vi "prompt_the_user_but_do_not_linger_v1.0.vi"() -> ()   [LabVIEW 2025]
doc: "Proof of concept/example VI for demonstration.\n\nMichael Panganiban\nSr. Hardware Test Engineer\nFresh Consulting, Inc."
uses:
  controls/home_navigation_btn.ctl
  controls/equipment_navigation_btn.ctl
  controls/settings_navigation_btn.ctl
  controls/test_plan_navigation_btn.ctl
panel:
  in  "test_plan":T1
  in  "settings":T2
  in  "equipment":T3
  in  "home":T4
  in  "Tab":T5(tab)
  out "start_of_test_status":string
  in  "start_test":bool
  # "v1.0.0.1"
  # "HOME"
  # "EQUIPMENT"
  # "SETTINGS"
  # "TEST PLAN CREATION"
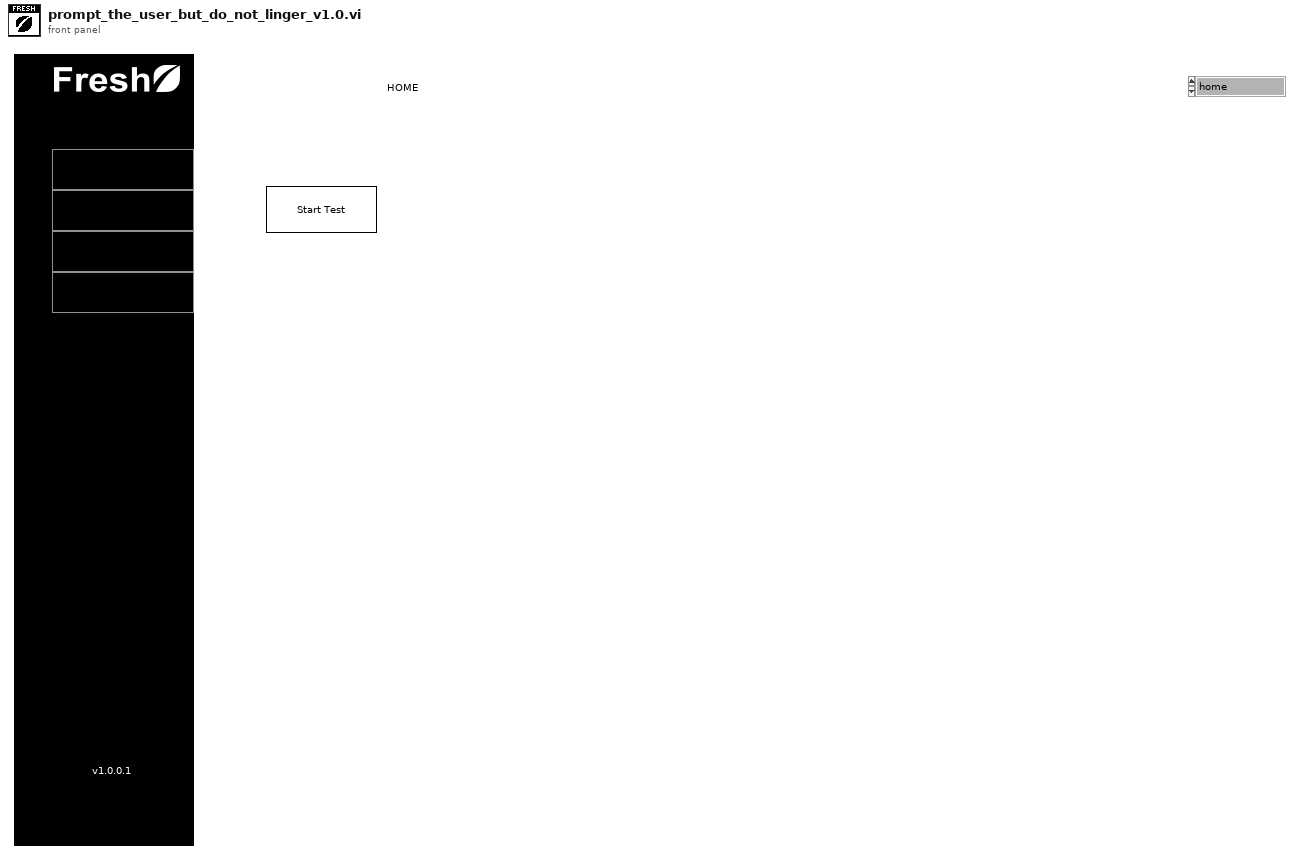
[diagram p1: front panel]
types:
  T1 = typedef "test_plan_navigation_btn.ctl" = bool
  T2 = typedef "settings_navigation_btn.ctl" = bool
  T3 = typedef "equipment_navigation_btn.ctl" = bool
  T4 = typedef "home_navigation_btn.ctl" = bool
  T5 = enum32{"home", "equipment", "settings", "test_plan"}
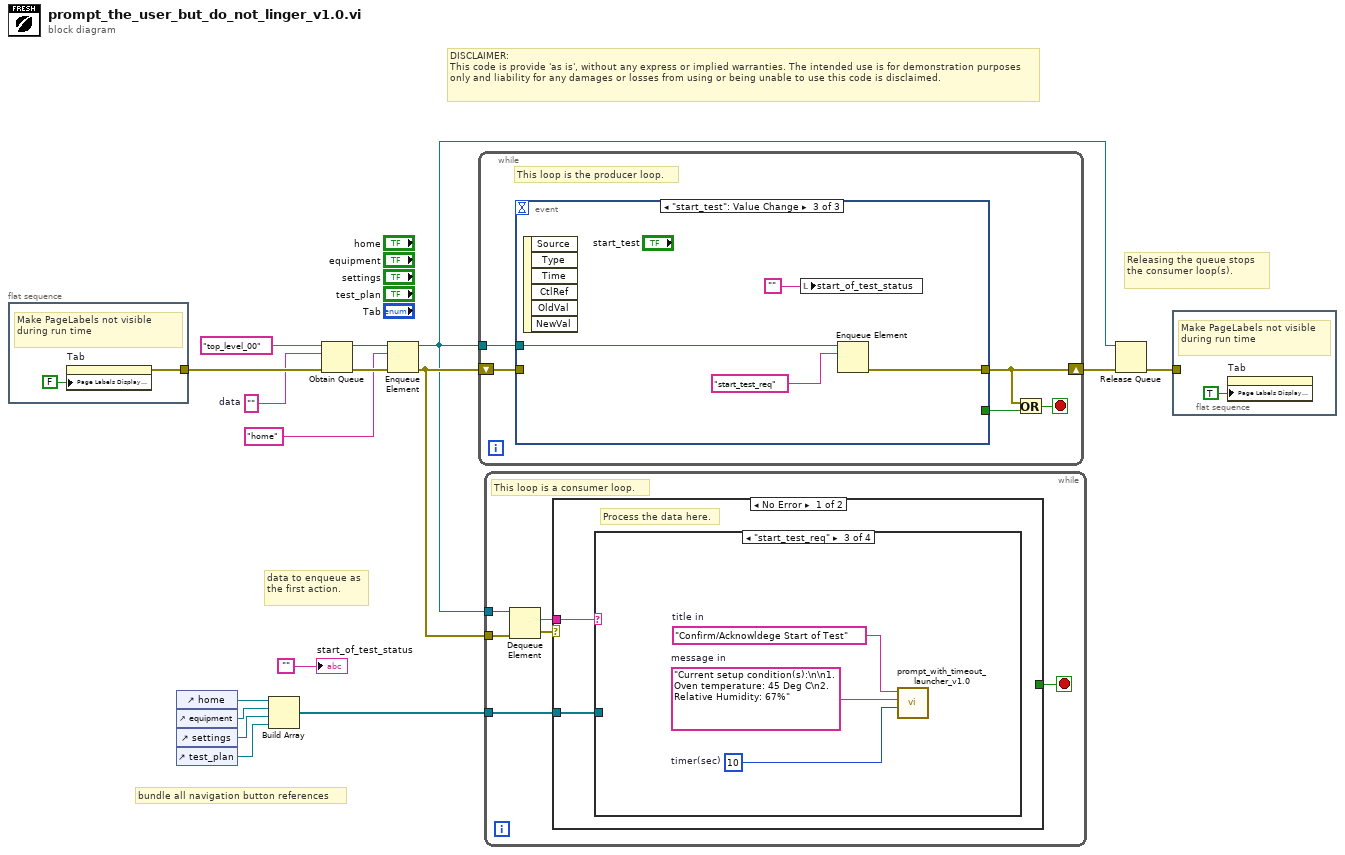
[diagram p0: block diagram]
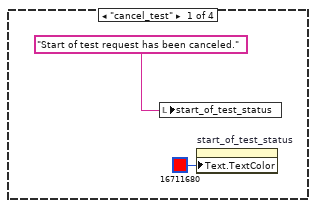
[diagram p2: hidden frame]
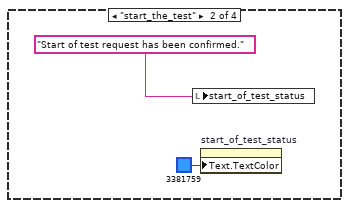
[diagram p3: hidden frame]
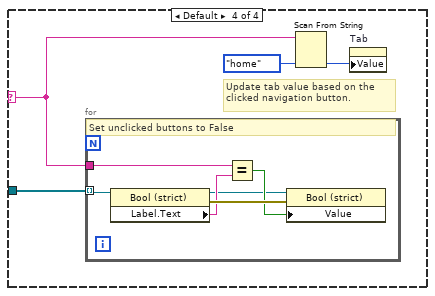
[diagram p4: hidden frame]
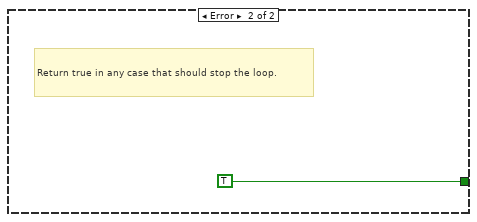
[diagram p5: hidden frame]
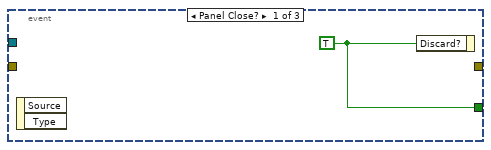
[diagram p6: hidden frame]
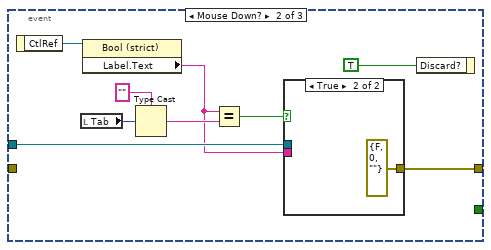
[diagram p7: hidden frame]
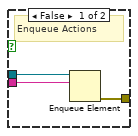
[diagram p8: hidden frame]
diagram:
  w2 = ""  # data
  # "data to enqueue as the first action."
  # "bundle all navigation button references"
  # "DISCLAIMER:\nThis code is provide 'as is', without any express or implied warranties. The intended use is for demonstration purposes only and liability for any damages or losses from using or being unable to use this code is disclaimed."
  # "Releasing the queue stops the consumer loop(s)."
  n1 = flat-sequence {
    tunnel: [w17] -> w15
    frame #0 {
      # "Make PageLabels not visible during run time"
      n2 = property on="Tab" class="TabCtl (strict)"("Page Labels Display Visible?"=FALSE) -> (error out=w17:errorcluster)  [unwired: 2 in, 1 out]
    }
  }
  n3 = control-ref of="home"() -> (w7:refnum<vi>)
  n4 = control-ref of="equipment"() -> (w13:refnum<vi>)
  n5 = control-ref of="settings"() -> (w12:refnum<vi>)
  n6 = control-ref of="test_plan"() -> (w11:refnum<vi>)
  n7 = Build Array(w7, w13, w12, w11) -> (w10:refnum<vi>[])
  n8 = Obtain Queue(name (unnamed)="top_level_00", element data type=w2, error in (no error)=w15) -> (queue out=w9:refnum<queue>, error out=w8:errorcluster)  [unwired: 2 in, 1 out]
  n9 = Enqueue Element(queue=w9, element="home" ("Action"), error in (no error)=w8) -> (queue out=w5:refnum<queue>, error out=w6:errorcluster)  [unwired: 1 in, 1 out]
  n10 = while {
    shift-right: [w20] -> w16
    shift-left: w6 -> [w23]
    tunnel: w5 -> [w19]
    stop <- w21 stop-if-true
    # "This loop is the producer loop."
    n11 = event shown="[2] \"start_test\": Value Change" {
      selector: _ -> [_ _ _]
      dyn-events: _ -> [_ _ _]
      timeout: _ -> [_ _ _]
      tunnel: w19 -> [_ w32 w41]
      tunnel: w23 -> [_ _ _]
      tunnel: [_ w33 w40] -> w20
      tunnel: [w24 _ _] -> w22
      event Panel Close? {
        w24 = TRUE ("Discard?")
        n12 = event-data() -> ()  [unwired: 1 in, 2 out]
        n13 = event-data("Discard?"=w24) -> ()  [unwired: 1 in, 1 out]
      }
      event Mouse Down? {
        n14 = event-data() -> ("CtlRef"=w31:refnum<vi>)  [unwired: 1 in]
        n15 = local read "Tab"() -> (w29:T5)
        n16 = property class="Bool (strict)"(reference=w31) -> ("Label.Text"=w25:string)  [unwired: 1 in, 2 out]
        n17 = Type Cast(type="", x=w29) -> (*(type *) &x=w27:string)
        n18 = Equal?(x=w25, y=w27) -> (x = y?=w26:bool)
        n19 = case shown="True" w26 {
          tunnel: [w36 errorcluster {"status"=FALSE, "code"=0, "source"=""} ("error out")] -> w33
          tunnel: w32 -> [w35 _]
          tunnel: w25 -> [w34 _]
          frame False {
            # "Enqueue Actions"
            n20 = Enqueue Element(queue=w35, element=w34) -> (error out=w36:errorcluster)  [unwired: 2 in, 2 out]
          }
          frame True {
          }
        }
        n21 = event-data("Discard?"=TRUE) -> ()  [unwired: 1 in, 1 out]
      }
      event "start_test": Value Change {
        n22 = event-data() -> ()  [unwired: 1 in, 6 out]
        n23 = local write "start_of_test_status"("") -> ()
        n24 = Enqueue Element(queue=w41, element="start_test_req" ("Action")) -> (error out=w40:errorcluster)  [unwired: 2 in, 2 out]
      }
    }
    n25 = Or(x=w20, y=w22) -> (x .or. y?=w21:bool)
  }
  n26 = while {
    tunnel: w5 -> [w47]
    tunnel: w10 -> [w43]
    tunnel: w6 -> [w42]
    stop <- w44 stop-if-true
    # "This loop is a consumer loop."
    n27 = Dequeue Element(queue=w47, error in (no error)=w42) -> (element=w45:string, error out=w46:errorcluster)  [unwired: 1 in, 2 out]
    n28 = case shown="No Error" w46 {
      tunnel: w45 -> [w48 _]
      tunnel: [_ TRUE] -> w44
      tunnel: w43 -> [w49 _]
      frame No Error {
        # "Process the data here."
        n29 = case shown="\"start_test_req\"" w48 {
          selector: w48 -> [_ _ _ w57]
          tunnel: w49 -> [_ _ _ w58]
          frame "cancel_test" {
            n30 = local write "start_of_test_status"("Start of test request has been canceled.") -> ()
            n31 = property on="start_of_test_status" class="Str"("Text.TextColor"=u32 16711680 ("Text.Text Colors:Text Color")) -> ()  [unwired: 2 in, 2 out]
          }
          frame "start_the_test" {
            n32 = local write "start_of_test_status"("Start of test request has been confirmed.") -> ()
            n33 = property on="start_of_test_status" class="Str"("Text.TextColor"=u32 3381759 ("Text.Text Colors:Text Color")) -> ()  [unwired: 2 in, 2 out]
          }
          frame "start_test_req" {
            w54 = 10  # timer(sec)
            w55 = "Current setup condition(s):\n\n1. Oven temperature: 45 Deg C\n2. Relative Humidity: 67%"  # message in
            w56 = "Confirm/Acknowldege Start of Test"  # title in
            n34 = call "prompt_with_timeout_launcher_v1.0.vi"("timer(sec)"=w54, "message in"=w55, "title in"=w56) -> ()  [unwired: 8 in, 1 out]
          }
          frame Default {
            # "Update tab value based on the clicked navigation button."
            n35 = for {
              tunnel: w58 -> [w66] mode=indexing
              tunnel: w57 -> [w63]
              # "Set unclicked buttons to False"
              n36 = property class="Bool (strict)"(reference=w66) -> (reference out=w61:refnum<vi>, error out=w65:errorcluster, "Label.Text"=w64:string)  [unwired: 1 in]
              n37 = Equal?(x=w63, y=w64) -> (x = y?=w62:bool)
              n38 = property class="Bool (strict)"(reference=w61, error in=w65, "Value"=w62) -> ()  [unwired: 2 out]
            }
            n39 = Scan From String(input string=w57, default 1=T5."home" ("Tab Control")) -> (output 1=w59:T5)  [unwired: 3 in, 3 out]
            n40 = property on="Tab" class="TabCtl (strict)"("Value"=w59) -> ()  [unwired: 2 in, 2 out]
          }
        }
      }
      frame Error {
        # "Return true in any case that should stop the loop."
      }
    }
  }
  n41 = Release Queue(queue=w5, error in (no error)=w16) -> (error out=w14:errorcluster)  [unwired: 1 in, 2 out]
  n42 = flat-sequence {
    tunnel: w14 -> [_]
    frame #0 {
      # "Make PageLabels not visible during run time"
      n43 = property on="Tab" class="TabCtl (strict)"("Page Labels Display Visible?"=TRUE) -> ()  [unwired: 2 in, 2 out]
    }
  }
  "start_of_test_status" <- ""
